vi "Periodic Tasks.vi"(8 "error in":errorcluster) -> ()   [LabVIEW 2019]
doc: "This VI runs in parallel to other tasks. It can contain as many user-defined periodic loops as you need. These can carry out PID or other sorts of timed response."
uses:
  <vilib>/Rock Robotics/WPI/ThirdParty/Sensors/navX/_TypeDefs/FRIC_navX_DeviceNumbersTypeDef.ctl
  <vilib>/Rock Robotics/WPI/DriverStation/WPI_DriverStationRobotMode2.ctl
  <vilib>/Rock Robotics/WPI/Solenoid/WPI_SolenoidValue.ctl
  <vilib>/Rock Robotics/WPI/Relay/WPI_RelayValue.ctl
  <vilib>/Rock Robotics/WPI/ThirdParty/Phoenix-LabVIEW/Motor Controller/Controls/CTRE_Phoenix_MotorControl_ControlMode.ctl
  LabVIEW_is_Under_Control.lib/Util/Toggle/Change Detect.vi
  LabVIEW_is_Under_Control.lib/Util/Toggle/Change Detect Boolean.vi
  MotorsGlobal.vi
  <vilib>/Rock Robotics/Network Tables/NT Read Number.vi
  <vilib>/Rock Robotics/WPI/Utilities/WPI_GetSetVariantRefNum.vi
  Robot Global Data.vi
  JoysticksGlobal.vi
  <vilib>/Rock Robotics/Network Tables/NT Write Number.vi
  <vilib>/Rock Robotics/WPI/Solenoid/WPI_SolenoidSetEnum.vi
  Ball Routine.ctl
  TurretMode.ctl
  <vilib>/Rock Robotics/WPI/ThirdParty/Phoenix-LabVIEW/Motor Controller/Controls/CTRE_Phoenix_MotorControl_FeedbackDevice.ctl
  Climber Routine.ctl
  <vilib>/Rock Robotics/WPI/ThirdParty/Phoenix-LabVIEW/Motor Controller/Get/CTRE_Phoenix_MotorController_GetVoltage.vi
  <vilib>/Rock Robotics/WPI/ThirdParty/Phoenix-LabVIEW/Motor Controller/Get/CTRE_Phoenix_MotorController_GetSelectedSensorData.vi
panel:
  in  "OutRoller":dbl=-0.8
  in  "OutShooter":dbl=0.6
  in  "OutConveyorRight":dbl=-0.1
  in  "OutConveyorMid":dbl=0.5
  in  "Setpoint Climber":dbl
  in  "OutIntake":dbl=0.6
  in  "OutConveyorLeft":dbl=-1.0
  out "Encoder Out":dbl
  in  "PIDs Tab":T1(tab)
  out "Current Intake":dbl
  in  "Reset Encoders":bool
  out "Current":dbl
  out "Motor Temperature":u8
  out "Current 2":dbl
  out "Motor Temperature 2":u8
  out "Current 3":dbl
  out "Motor Temperature 3":u8
  out "Current 4":dbl
  out "Motor Temperature 4":u8
  out "Current Intake 2":dbl
  out "Current Intake 3":dbl
  in  "MaxAngle":dbl
  out "LimelightX":dbl
  out "Turret PID":cluster{"Setpoint":dbl, "Process variable":dbl}(graph)
  in  "Camera Angle":dbl=7.0
  out "Distancia do Goal":dbl
  in  "Inner Goal Height":dbl=2.49
  in  "Camera Height":dbl=0.185
  in  "Minimum command":dbl=0.031
  out "Turret Out":dbl
  in  "TAGains":T2={"proportional gain (Kc)"=1.0, "integral time (Ti, min)"=0.01, "derivative time (Td, min)"=0.0} {"derivative time (Td, min)" format="%.3f"; "integral time (Ti, min)" format="%.3f"; "proportional gain (Kc)" format="%.3f"}
  in  "TADisable Range":dbl
  in  "TAIntegral Range":dbl=10000.0
  in  "TASetpoint":dbl
  in  "TARange":cluster{"output high":dbl, "output low":dbl}={"output high"=0.6, "output low"=-0.6} {"output low" format="%.2f"; "output high" format="%.2f"}
  out "Voltage":dbl
  out "Voltage Output":cluster{"Percent Output":dbl}(graph)
  out "Velocity PIDF":T3(graph)
  in  "kF":dbl=0.031
  in  "EnableFWPID":bool
  in  "FWSetpoint":dbl
  in  "P":dbl
  in  "I":dbl
  in  "D":dbl
  in  "I Zone":dbl
  # "System Tester"
  # "Sparks Max"
  # "ID-1"
  # "ID-2"
  # "ID-3"
  # "ID-4"
  # "Distance Meter"
  # "All in cm"
  # "Turret Angle PID"
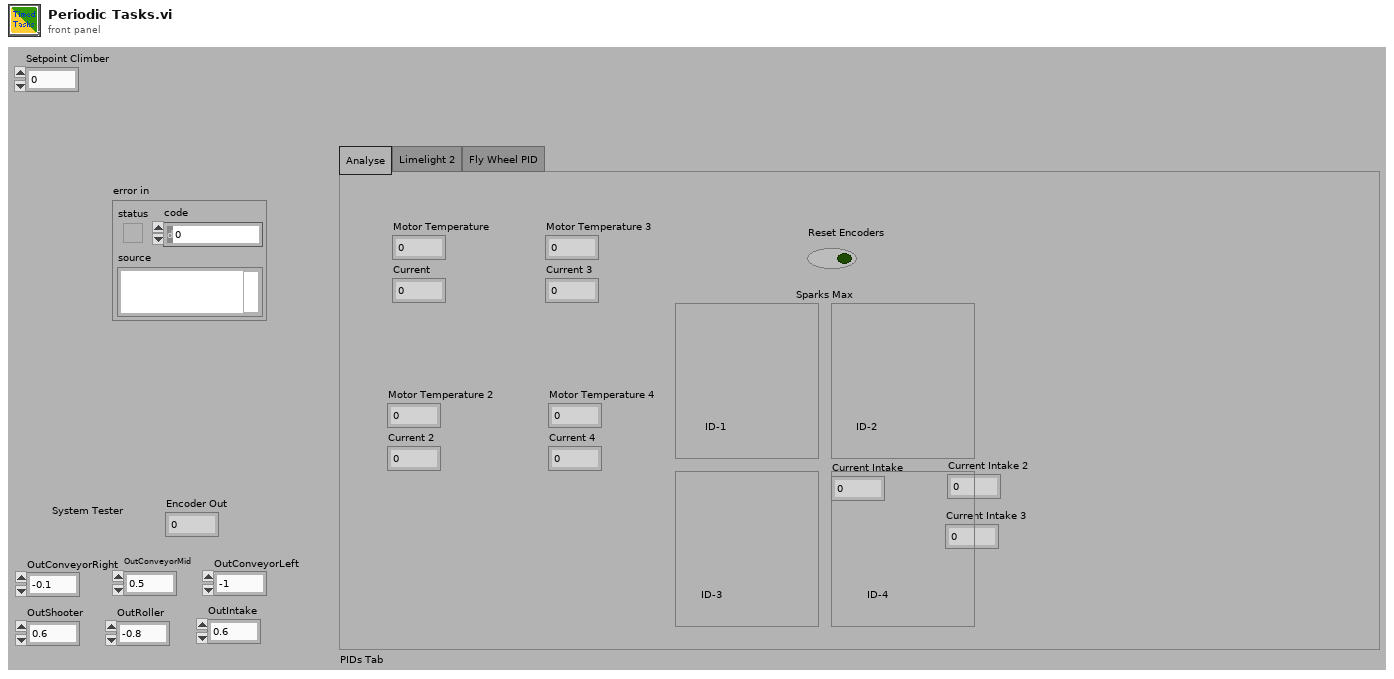
[diagram p1: front panel]
types:
  T1 = enum32{"Analyse", "Limelight 2", "Fly Wheel PID"}
  T2 = cluster{"proportional gain (Kc)":dbl, "integral time (Ti, min)":dbl, "derivative time (Td, min)":dbl}
  T3 = cluster{"FWSetpoint":dbl, "Velocity (Raw Sensor Units per 100 ms)":i32}
  T4 = typedef "WPI_EncoderDevRef.ctl" = cluster{"DevStatus":errorcluster, "EncoderIndex":T5, "CounterIndex":T6, "DistancePerCount":dbl, "Decoding Type":T7}
  T5 = typedef "FPGA_EncoderIdx.ctl" = enum8{"Enc 0", "Enc 1", "Enc 2", "Enc 3", "Enc 4", "Enc 5", "Enc 6", "Enc 7", "Invalid"}
  T6 = typedef "FPGA_CounterCtrSystemIndex.ctl" = enum8{"Ctr 0", "Ctr 1", "Ctr 2", "Ctr 3", "Ctr 4", "Ctr 5", "Ctr 6", "Ctr 7", "Invalid"}
  T7 = typedef "WPI_EncoderType.ctl" = enum16{"1x", "2x", "4x"}
  T8 = typedef "WPI_SwitchDevRef.ctl" = cluster{"DevStatus":errorcluster, "DIO Channel":T9, "CntIndex":T6, "Normally Closed":bool}
  T9 = typedef "FPGA_DIOChannel.ctl" = enum8{"DIO 0", "DIO 1", "DIO 2", "DIO 3", "DIO 4", "DIO 5", "DIO 6", "DIO 7", "DIO 8", "DIO 9", "DIO MXP 0", "DIO MXP 1", "DIO MXP 2", "DIO MXP 3", "DIO MXP 4", "DIO MXP 5", "DIO MXP 6", "DIO MXP 7", "DIO MXP 8", "DIO MXP 9", "DIO MXP 10", "DIO MXP 11", "DIO MXP 12", "DIO MXP 13", "DIO MXP 14", "DIO MXP 15", "SPI Port CS1", "SPI Port CS2", "SPI Port CS3", "SPI Port MISO", "SPI Port MOSI", "Invalid"}
  T10 = typedef "FRIC_navX_DeviceNumbersTypeDef.ctl" = enum16{"Dev0", "Dev1", "Dev2", "Dev3"}
  T11 = cluster{"Rollover":dbl, "Yaw":dbl, "Cont Yaw":dbl}
  T12 = typedef "WPI_MotorControlDeviceRef.ctl" = cluster{"DeviceStatus":errorcluster, "Type":T13, "PWM":cluster{"PWM Channel":T14, "DeadBand":T15}, "CAN":cluster{"Device Number":u8, "SetOutput VI Ref":variant, "GetOutput VI Ref":variant, "Enable VI Ref":variant, "Disable VI Ref":variant, "Data":variant}, "Invert":bool, "DIO PWM":cluster{"PWM \"Enable\" Channel":T14, "DIOChannel":T9, "PWM Rate":dbl}}
  T13 = typedef "WPI_MotorControlType.ctl" = enum16{"PWM", "CAN", "DIO PWM"}
  T14 = typedef "FPGA_DIOPWMChannel.ctl" = enum8{"PWM 0", "PWM 1", "PWM 2", "PWM 3", "PWM 4", "PWM 5", "PWM 6", "PWM 7", "PWM 8", "PWM 9", "PWM MXP 0", "PWM MXP 1", "PWM MXP 2", "PWM MXP 3", "PWM MXP 4", "PWM MXP 5", "PWM MXP 6", "PWM MXP 7", "PWM MXP 8", "PWM MXP 9", "Invalid"}
  T15 = typedef "WPI_PWMDeadband.ctl" = cluster{"Name":string, "maxPositivePwm":i32, "minPositivePwm":i32, "centerPwm":i32, "maxNegativePwm":i32, "minNegativePwm":i32, "angularRange":u16}
  T16 = typedef "WPI_JoystickDevRef.ctl" = cluster{"Device":T17}
  T17 = typedef "WPI_JoystickDeviceEnum.ctl" = enum16{"USB 0", "USB 1", "USB 2", "USB 3", "USB 4", "USB 5"}
  T18 = typedef "WPI_SolenoidDevRef.ctl" = cluster{"DevStatus":errorcluster, "Pneumatics Control Module":u8, "Forward Solenoid Channel":T19, "Reverse Solenoid Channel":T19}
  T19 = typedef "WPI_SolenoidChannel.ctl" = enum8{"Solenoid 0", "Solenoid 1", "Solenoid 2", "Solenoid 3", "Solenoid 4", "Solenoid 5", "Solenoid 6", "Solenoid 7", "Invalid"}
  T20 = typedef "WPI_RelayDevRef.ctl" = cluster{"DevStatus":errorcluster, "Relay Channel":T21, "Relay Direction":T22}
  T21 = typedef "FPGA_DIORelayChannel.ctl" = enum8{"Relay 0", "Relay 1", "Relay 2", "Relay 3", "Invalid"}
  T22 = typedef "WPI_RelayDirection.ctl" = enum16{"Both directions", "Forward only", "Reverse only"}
  T23 = typedef "WPI_RelayValue.ctl" = enum16{"Off", "On", "Forward", "Reverse"}
  T24 = typedef "WPI_SolenoidValue.ctl" = enum16{"Off", "On", "Forward", "Reverse"}
  T25 = typedef "CTRE_Phoenix_MotorControl_ControlMode.ctl" = u16
  T26 = typedef "WPI_DriverStationRobotMode2.ctl" = enum16{"Autonomous Disabled", "Autonomous Enabled", "Teleop Disabled", "Teleop Enabled", "Disconnected", "Finish", "Test Disabled", "Test Enabled", "Emergency Stopped"}
  T27 = typedef "WPI_RobotDriveDevRef.ctl" = cluster{"DevStatus":errorcluster, "Motors[]":T12[], "Square Inputs":bool, "Max Output":dbl}
  T28 = cluster{"Motors[][0]":T12, "Motors[][1]":T12, "Motors[][2]":T12, "Motors[][3]":T12, "Motors[][4]":T12, "Motors[][5]":T12, "Motors[][6]":T12, "Motors[][7]":T12, "Motors[][8]":T12}
  T29 = typedef "Climber Routine.ctl" = enum16{"Standart", "Vibrate *Lenny Face*", "Open da Boi", "Engage on the Bar!", "Pull Our Hope", "Deu por Hoje"}
  T30 = typedef "TurretMode.ctl" = enum16{"Static", "Manual", "Automatic"}
  T31 = typedef "Ball Routine.ctl" = enum16{"Standart", "Get Power Cells", "Prepare Shooter", "Shoot!"}
  T32 = typedef "CTRE_Phoenix_MotorControl_FeedbackDevice.ctl" = i8
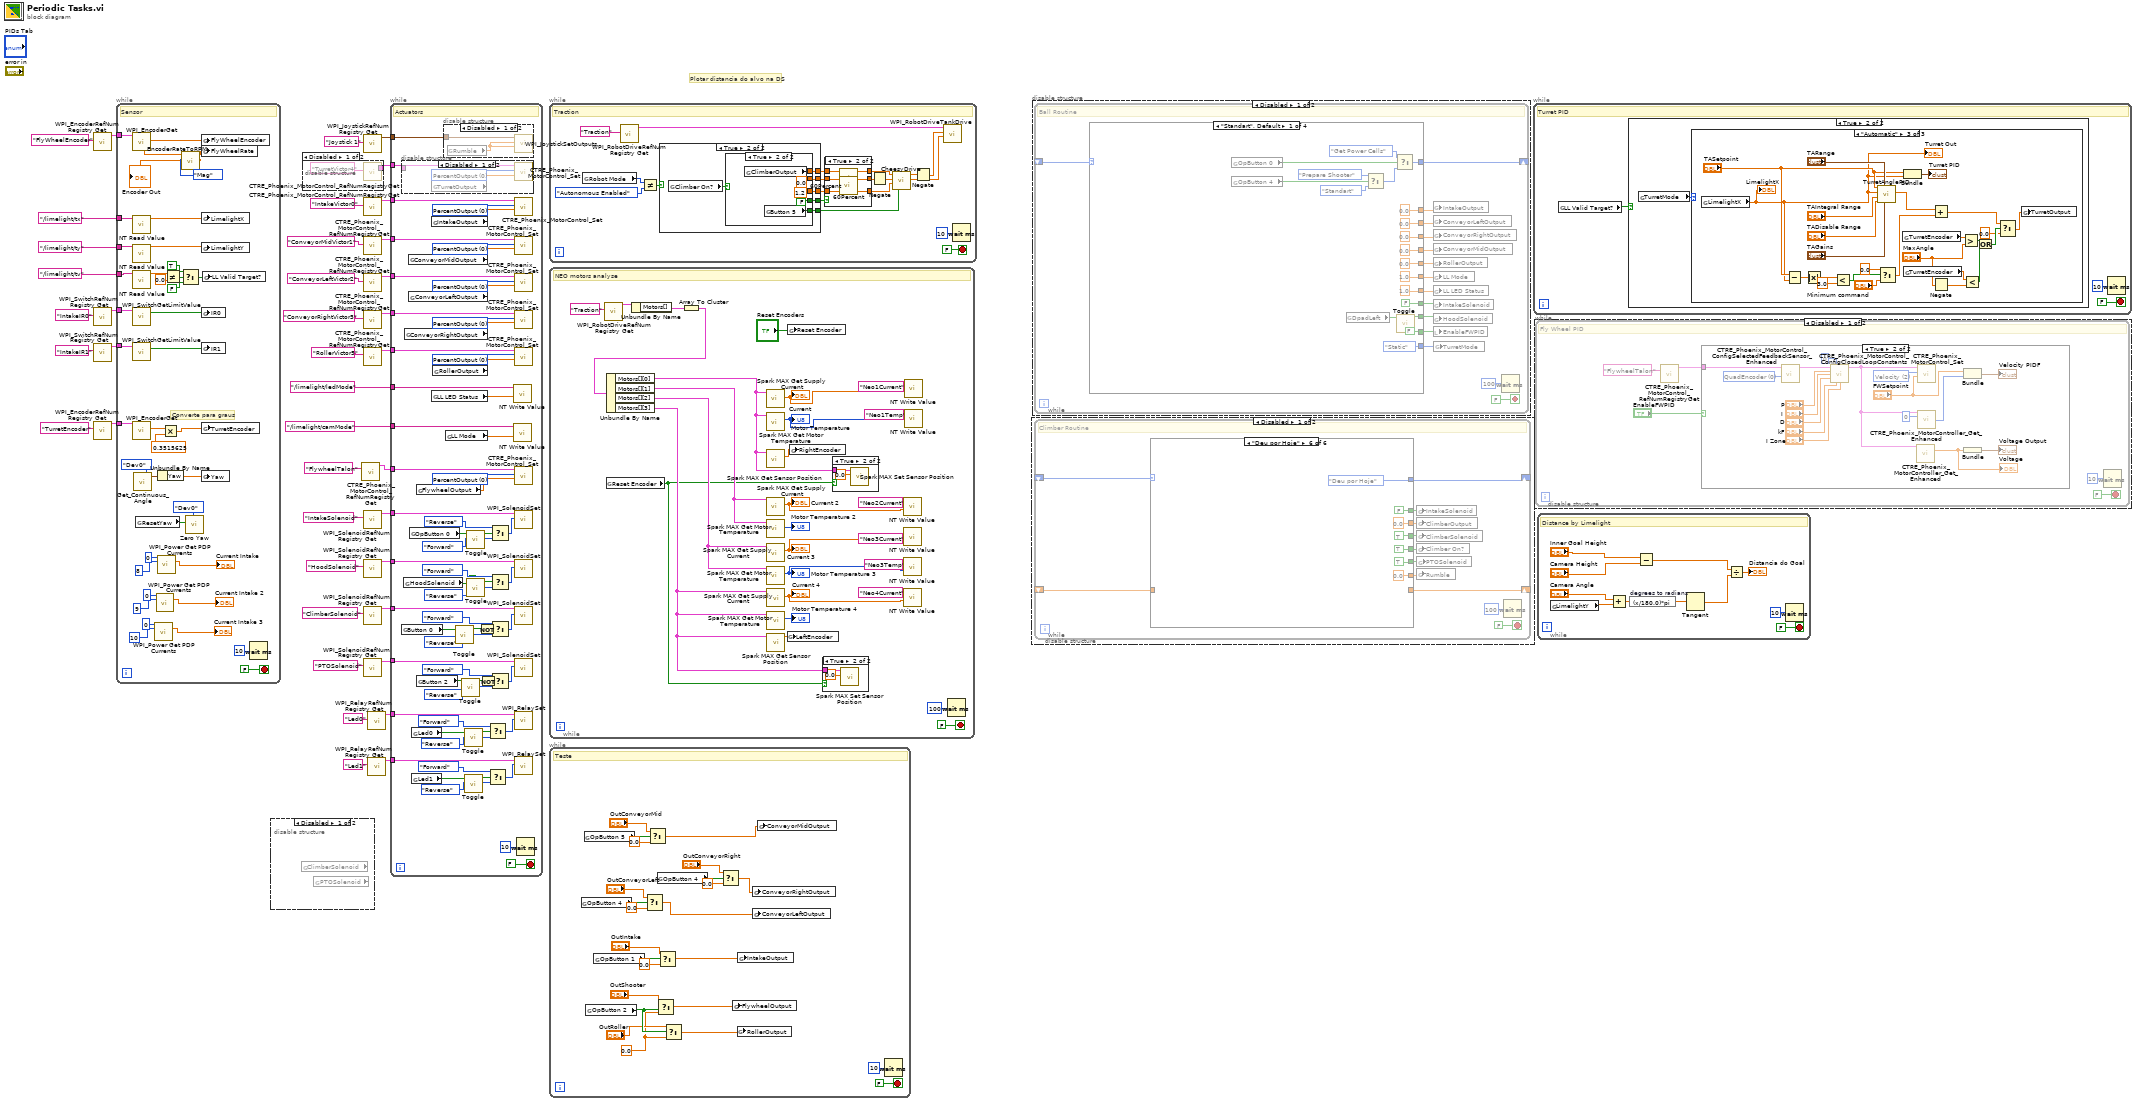
[diagram p0: block diagram]
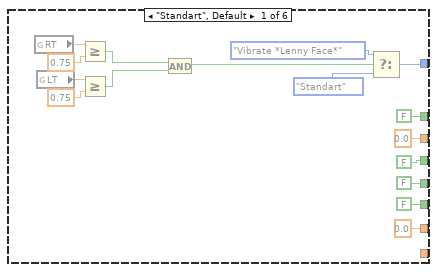
[diagram p2: hidden frame]
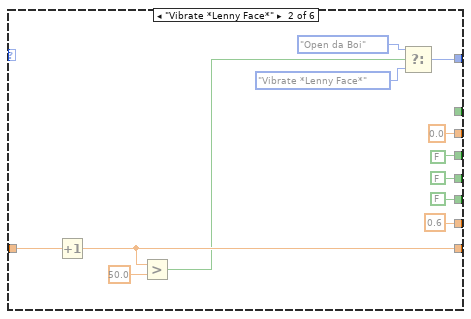
[diagram p3: hidden frame]
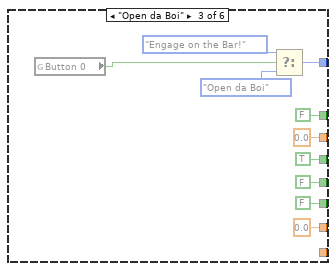
[diagram p4: hidden frame]
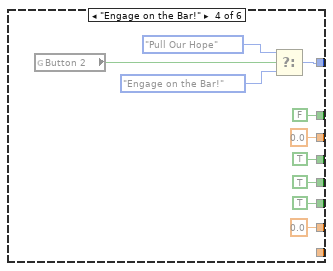
[diagram p5: hidden frame]
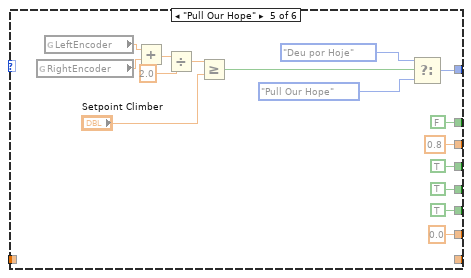
[diagram p6: hidden frame]
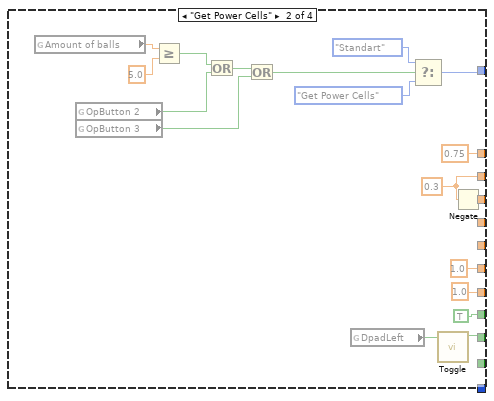
[diagram p10: hidden frame]
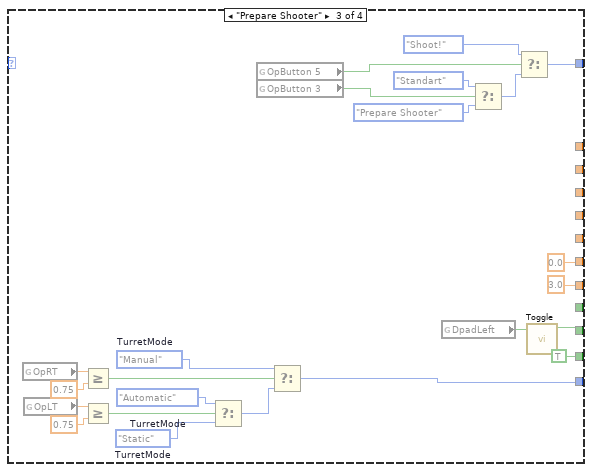
[diagram p11: hidden frame]
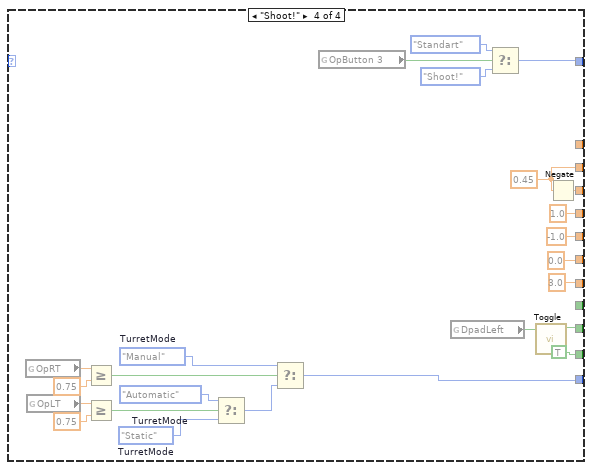
[diagram p12: hidden frame]
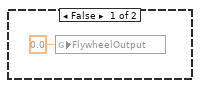
[diagram p14: hidden frame]
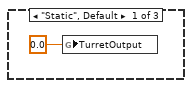
[diagram p19: hidden frame]
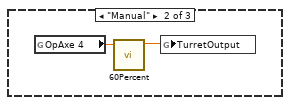
[diagram p20: hidden frame]
diagram:
  # "Plotar distancia do alvo na DS"
  n1 = call <vilib>:"WPI_EncoderRefNum Registry Get.vi"("refnum name"="FlyWheelEncoder") -> ("EncoderDevRef"=w40:T4)  [unwired: 9 in, 1 out]
  n2 = call <vilib>:"WPI_SwitchRefNum Registry Get.vi"("refnum name"="IntakeIR0") -> ("SwitchDevRef"=w23:T8)  [unwired: 9 in, 1 out]
  n3 = call <vilib>:"WPI_SwitchRefNum Registry Get.vi"("refnum name"="IntakeIR1") -> ("SwitchDevRef"=w20:T8)  [unwired: 9 in, 1 out]
  n4 = call <vilib>:"WPI_EncoderRefNum Registry Get.vi"("refnum name"="TurretEncoder") -> ("EncoderDevRef"=w15:T4)  [unwired: 9 in, 1 out]
  n5 = while {
    tunnel: w40 -> [w79]
    tunnel: "/limelight/tx" ("Name") -> [w73]
    tunnel: "/limelight/ty" ("Name") -> [w70]
    tunnel: w23 -> [w69]
    tunnel: w20 -> [w66]
    tunnel: "/limelight/tv" ("Name") -> [w65]
    tunnel: w15 -> [w58]
    stop <- FALSE stop-if-true
    # "Converte para graus"
    # "Sensor"
    n6 = call <vilib>:"WPI_EncoderGet.vi"("EncoderDevRef"=w79) -> ("Distance"=w77:dbl, "Rate"=w76:dbl)  [unwired: 5 in, 4 out]
    n7 = call-poly <vilib>:"NT Read Value.vi"("Name"=w73) -> ("Numeric"=w72:dbl)  [unwired: 9 in, 1 out]
    n8 = call-poly <vilib>:"NT Read Value.vi"("Name"=w70) -> ("Numeric"=w71:dbl)  [unwired: 9 in, 1 out]
    n9 = call-poly <vilib>:"NT Read Value.vi"("Name"=w65) -> ("Numeric"=w64:dbl)  [unwired: 9 in, 1 out]
    n10 = call <vilib>:"WPI_SwitchGetLimitValue.vi"("SwitchDevRef"=w69) -> ("Switch Pressed"=w68:bool)  [unwired: 8 in, 2 out]
    n11 = call <vilib>:"WPI_SwitchGetLimitValue.vi"("SwitchDevRef"=w66) -> ("Switch Pressed"=w67:bool)  [unwired: 8 in, 2 out]
    n12 = call <vilib>:"WPI_EncoderGet.vi"("EncoderDevRef"=w58) -> ("Distance"=w57:dbl)  [unwired: 5 in, 5 out]
    n13 = call <vilib>:"Get_Continuous_Angle.vi"("Device Number"=FRIC_navX_DeviceNumbersTypeDef."Dev0") -> ("Continuous Angle"=w53:T11)  [unwired: 10 in]
    n14 = global read "MotorsGlobal.vi" "ResetYaw"() -> (w50:bool)
    n15 = call <vilib>:"WPI_Power Get PDP Currents.vi"("Power Distribution Panel (0)"=u8 0, "PDP Channel"=10) -> ("current (A)"=→"Current Intake 3":dbl)  [unwired: 11 in, 2 out]
    n16 = call <vilib>:"WPI_Power Get PDP Currents.vi"("Power Distribution Panel (0)"=u8 0, "PDP Channel"=9) -> ("current (A)"=→"Current Intake 2":dbl)  [unwired: 11 in, 2 out]
    n17 = call <vilib>:"WPI_Power Get PDP Currents.vi"("Power Distribution Panel (0)"=u8 0, "PDP Channel"=8) -> ("current (A)"=→"Current Intake":dbl)  [unwired: 11 in, 2 out]
    n18 = Unbundle By Name(w53) -> ("Yaw"=w52:dbl)
    n19 = Multiply(x=w57, y=0.3515625) -> (x*y=w55:dbl)
    n20 = Not Equal?(x=w64, y=0.0) -> (x != y?=w62:bool)
    n21 = call "EncoderRateToRPM.vi"("Enum"=enum16{"Through Bore", "Mag"}."Mag", "EncoderRate"=w76) -> ("RPM"=→"Encoder Out":dbl, "RPS"=w75:dbl)  [unwired: 8 in]
    n22 = Select(t=TRUE, s=w62, f=FALSE) -> (s? t:f=w61:bool)
    n23 = call <vilib>:"Zero Yaw.vi"("Device Number"=FRIC_navX_DeviceNumbersTypeDef."Dev0", "Zero"=w50) -> ()  [unwired: 10 in]
    n24 = global write "MotorsGlobal.vi" "FlyWheelEncoder"(w77) -> ()
    n25 = global write "MotorsGlobal.vi" "FlyWheelRate"(w75) -> ()
    n26 = global write "MotorsGlobal.vi" "LimelightX"(w72) -> ()
    n27 = global write "MotorsGlobal.vi" "LimelightY"(w71) -> ()
    n28 = global write "MotorsGlobal.vi" "IR0"(w68) -> ()
    n29 = global write "MotorsGlobal.vi" "IR1"(w67) -> ()
    n30 = global write "MotorsGlobal.vi" "Yaw"(w52) -> ()
    n31 = global write "MotorsGlobal.vi" "TurretEncoder"(w55) -> ()
    n32 = global write "MotorsGlobal.vi" "LL Valid Target?"(w61) -> ()
    n33 = Wait (ms)(milliseconds to wait=u32 10) -> ()  [unwired: 1 out]
  }
  n34 = disable-structure shown="Disabled" {
    frame Disabled {
      n35 = global read "MotorsGlobal.vi" "ClimberSolenoid"() -> ()  [unwired: 1 out]
      n36 = global read "MotorsGlobal.vi" "PTOSolenoid"() -> ()  [unwired: 1 out]
    }
    frame Enabled {
    }
  }
  n37 = disable-structure shown="Disabled" {
    disable-tunnel: [w83 _] -> w36
    frame Disabled {
      n38 = call <vilib>:"CTRE_Phoenix_MotorControl_RefNumRegistryGet.vi"("refnum name"="TurretVictor4") -> ("PhoenixMotorControlDevRef"=w83:T12)  [unwired: 9 in, 1 out]
    }
    frame Enabled {
    }
  }
  n39 = call <vilib>:"CTRE_Phoenix_MotorControl_RefNumRegistryGet.vi"("refnum name"="FlywheelTalon") -> ("PhoenixMotorControlDevRef"=w1:T12)  [unwired: 9 in, 1 out]
  n40 = call <vilib>:"WPI_JoystickRefNum Registry Get.vi"("refnum name"="Joystick 1") -> ("JoystickDevRef"=w13:T16)  [unwired: 9 in, 1 out]
  n41 = call <vilib>:"CTRE_Phoenix_MotorControl_RefNumRegistryGet.vi"("refnum name"="IntakeVictor0") -> ("PhoenixMotorControlDevRef"=w35:T12)  [unwired: 9 in, 1 out]
  n42 = call <vilib>:"CTRE_Phoenix_MotorControl_RefNumRegistryGet.vi"("refnum name"="ConveyorMidVictor1") -> ("PhoenixMotorControlDevRef"=w34:T12)  [unwired: 9 in, 1 out]
  n43 = call <vilib>:"CTRE_Phoenix_MotorControl_RefNumRegistryGet.vi"("refnum name"="ConveyorLeftVictor2") -> ("PhoenixMotorControlDevRef"=w33:T12)  [unwired: 9 in, 1 out]
  n44 = call <vilib>:"CTRE_Phoenix_MotorControl_RefNumRegistryGet.vi"("refnum name"="ConveyorRightVictor3") -> ("PhoenixMotorControlDevRef"=w32:T12)  [unwired: 9 in, 1 out]
  n45 = call <vilib>:"CTRE_Phoenix_MotorControl_RefNumRegistryGet.vi"("refnum name"="RollerVictor5") -> ("PhoenixMotorControlDevRef"=w24:T12)  [unwired: 9 in, 1 out]
  n46 = call <vilib>:"WPI_SolenoidRefNum Registry Get.vi"("refnum name"="IntakeSolenoid") -> ("SolenoidDevRef"=w30:T18)  [unwired: 9 in, 1 out]
  n47 = call <vilib>:"WPI_SolenoidRefNum Registry Get.vi"("refnum name"="HoodSolenoid") -> ("SolenoidDevRef"=w27:T18)  [unwired: 9 in, 1 out]
  n48 = call <vilib>:"WPI_SolenoidRefNum Registry Get.vi"("refnum name"="ClimberSolenoid") -> ("SolenoidDevRef"=w26:T18)  [unwired: 9 in, 1 out]
  n49 = call <vilib>:"WPI_SolenoidRefNum Registry Get.vi"("refnum name"="PTOSolenoid") -> ("SolenoidDevRef"=w11:T18)  [unwired: 9 in, 1 out]
  n50 = call <vilib>:"WPI_RelayRefNum Registry Get.vi"("refnum name"="Led0") -> ("RelayDevRef"=w9:T20)  [unwired: 9 in, 1 out]
  n51 = call <vilib>:"WPI_RelayRefNum Registry Get.vi"("refnum name"="Led1") -> ("RelayDevRef"=w8:T20)  [unwired: 9 in, 1 out]
  n52 = while {
    tunnel: w36 -> [w145]
    tunnel: w35 -> [w144]
    tunnel: w34 -> [w143]
    tunnel: w33 -> [w142]
    tunnel: w32 -> [w141]
    tunnel: w30 -> [w140]
    tunnel: w27 -> [w131]
    tunnel: w26 -> [w130]
    tunnel: w24 -> [w125]
    tunnel: "/limelight/ledMode" ("Name") -> [w124]
    tunnel: "/limelight/camMode" ("Name") -> [w121]
    tunnel: w13 -> [w120]
    tunnel: w11 -> [w115]
    tunnel: w9 -> [w114]
    tunnel: w8 -> [w103]
    tunnel: w1 -> [w86]
    stop <- FALSE stop-if-true
    w87 = T25 0 items=["PercentOutput"=0, "Position"=1, "Velocity"=2, "Current"=3, "Follower"=5, "MotionProfile"=6, "MotionMagic"=7, "MotionProfileArc"=10, "Disabled"=15] ("Control Mode")
    w89 = T25 0 items=["PercentOutput"=0, "Position"=1, "Velocity"=2, "Current"=3, "Follower"=5, "MotionProfile"=6, "MotionMagic"=7, "MotionProfileArc"=10, "Disabled"=15] ("Control Mode")
    w95 = T25 0 items=["PercentOutput"=0, "Position"=1, "Velocity"=2, "Current"=3, "Follower"=5, "MotionProfile"=6, "MotionMagic"=7, "MotionProfileArc"=10, "Disabled"=15] ("Control Mode")
    w97 = T25 0 items=["PercentOutput"=0, "Position"=1, "Velocity"=2, "Current"=3, "Follower"=5, "MotionProfile"=6, "MotionMagic"=7, "MotionProfileArc"=10, "Disabled"=15] ("Control Mode")
    w99 = T25 0 items=["PercentOutput"=0, "Position"=1, "Velocity"=2, "Current"=3, "Follower"=5, "MotionProfile"=6, "MotionMagic"=7, "MotionProfileArc"=10, "Disabled"=15] ("Control Mode")
    w102 = T25 0 items=["PercentOutput"=0, "Position"=1, "Velocity"=2, "Current"=3, "Follower"=5, "MotionProfile"=6, "MotionMagic"=7, "MotionProfileArc"=10, "Disabled"=15] ("Control Mode")
    # "Actuators"
    n53 = disable-structure shown="Disabled" {
      disable-tunnel: w145 -> [w152 _]
      frame Disabled {
        w151 = T25 0 items=["PercentOutput"=0, "Position"=1, "Velocity"=2, "Current"=3, "Follower"=5, "MotionProfile"=6, "MotionMagic"=7, "MotionProfileArc"=10, "Disabled"=15] ("Control Mode")
        n54 = global read "MotorsGlobal.vi" "TurretOutput"() -> (w150:dbl)
        n55 = call <vilib>:"CTRE_Phoenix_MotorControl_Set.vi"("Output"=w150, "Control Mode"=w151, "PhoenixMotorControlDevRef"=w152) -> ()  [unwired: 7 in, 2 out]
      }
      frame Enabled {
      }
    }
    n56 = global read "JoysticksGlobal.vi" "Button 0"() -> (w92:bool)
    n57 = global read "MotorsGlobal.vi" "HoodSolenoid"() -> (w93:bool)
    n58 = global read "MotorsGlobal.vi" "ConveyorRightOutput"() -> (w94:dbl)
    n59 = global read "MotorsGlobal.vi" "ConveyorMidOutput"() -> (w98:dbl)
    n60 = global read "MotorsGlobal.vi" "ConveyorLeftOutput"() -> (w96:dbl)
    n61 = global read "JoysticksGlobal.vi" "OpButton 0"() -> (w100:bool)
    n62 = global read "MotorsGlobal.vi" "Led0"() -> (w109:bool)
    n63 = global read "MotorsGlobal.vi" "Led1"() -> (w108:bool)
    n64 = global read "MotorsGlobal.vi" "FlywheelOutput"() -> (w88:dbl)
    n65 = global read "JoysticksGlobal.vi" "Button 2"() -> (w91:bool)
    n66 = global read "MotorsGlobal.vi" "IntakeOutput"() -> (w101:dbl)
    n67 = global read "MotorsGlobal.vi" "LL LED Status"() -> (w123:dbl)
    n68 = global read "MotorsGlobal.vi" "RollerOutput"() -> (w90:dbl)
    n69 = disable-structure shown="Disabled" {
      disable-tunnel: w120 -> [w149 _]
      frame Disabled {
        n70 = global read "JoysticksGlobal.vi" "Rumble"() -> (w148:dbl)
        n71 = call <vilib>:"WPI_JoystickSetOutputs.vi"("Right Rumble"=w148, "Left Rumble"=w148, "JoystickDevRef"=w149) -> ()  [unwired: 7 in, 2 out]
      }
      frame Enabled {
      }
    }
    n72 = global read "MotorsGlobal.vi" "LL Mode"() -> (w122:dbl)
    n73 = call "Toggle.vi"("In"=w92) -> ("Toggled"=w126:bool)  [unwired: 10 in]
    n74 = call "Toggle.vi"("In"=w91) -> ("Toggled"=w119:bool)  [unwired: 10 in]
    n75 = call "Toggle.vi"("In"=w109) -> ("Toggled"=w113:bool)  [unwired: 10 in]
    n76 = call "Toggle.vi"("In"=w108) -> ("Toggled"=w104:bool)  [unwired: 10 in]
    n77 = call "Toggle.vi"("In"=w100) -> ("Toggled"=w136:bool)  [unwired: 10 in]
    n78 = call "Toggle.vi"("In"=w93) -> ("Toggled"=w135:bool)  [unwired: 10 in]
    n79 = Not(x=w126) -> (.not. x?=w85:bool)
    n80 = Not(x=w119) -> (.not. x?=w84:bool)
    n81 = Select(t=WPI_RelayValue."Forward" ("RelayValue"), s=w113, f=WPI_RelayValue."Reverse" ("RelayValue")) -> (s? t:f=w112:T23)
    n82 = Select(t=WPI_RelayValue."Forward" ("RelayValue"), s=w104, f=WPI_RelayValue."Reverse" ("RelayValue")) -> (s? t:f=w105:T23)
    n83 = Select(t=WPI_SolenoidValue."Reverse" ("Value"), s=w136, f=WPI_SolenoidValue."Forward" ("Value")) -> (s? t:f=w138:T24)
    n84 = Select(t=WPI_SolenoidValue."Forward" ("Value"), s=w135, f=WPI_SolenoidValue."Reverse" ("Value")) -> (s? t:f=w133:T24)
    n85 = Select(t=WPI_SolenoidValue."Forward" ("Value"), s=w85, f=WPI_SolenoidValue."Reverse" ("Value")) -> (s? t:f=w128:T24)
    n86 = Select(t=WPI_SolenoidValue."Forward" ("Value"), s=w84, f=WPI_SolenoidValue."Reverse" ("Value")) -> (s? t:f=w117:T24)
    n87 = call-poly <vilib>:"NT Write Value.vi"("Numeric"=w123, "Name"=w124) -> ()  [unwired: 9 in, 1 out]
    n88 = call-poly <vilib>:"NT Write Value.vi"("Numeric"=w122, "Name"=w121) -> ()  [unwired: 9 in, 1 out]
    n89 = call <vilib>:"CTRE_Phoenix_MotorControl_Set.vi"("Output"=w101, "Control Mode"=w102, "PhoenixMotorControlDevRef"=w144) -> ()  [unwired: 7 in, 2 out]
    n90 = call <vilib>:"CTRE_Phoenix_MotorControl_Set.vi"("Output"=w98, "Control Mode"=w99, "PhoenixMotorControlDevRef"=w143) -> ()  [unwired: 7 in, 2 out]
    n91 = call <vilib>:"CTRE_Phoenix_MotorControl_Set.vi"("Output"=w96, "Control Mode"=w97, "PhoenixMotorControlDevRef"=w142) -> ()  [unwired: 7 in, 2 out]
    n92 = call <vilib>:"CTRE_Phoenix_MotorControl_Set.vi"("Output"=w94, "Control Mode"=w95, "PhoenixMotorControlDevRef"=w141) -> ()  [unwired: 7 in, 2 out]
    n93 = call <vilib>:"CTRE_Phoenix_MotorControl_Set.vi"("Output"=w90, "Control Mode"=w89, "PhoenixMotorControlDevRef"=w125) -> ()  [unwired: 7 in, 2 out]
    n94 = call <vilib>:"CTRE_Phoenix_MotorControl_Set.vi"("Output"=w88, "Control Mode"=w87, "PhoenixMotorControlDevRef"=w86) -> ()  [unwired: 7 in, 2 out]
    n95 = call-poly <vilib>:"WPI_SolenoidSet.vi"("Value"=w138, "SolenoidDevRef"=w140) -> ()  [unwired: 8 in, 2 out]
    n96 = call-poly <vilib>:"WPI_SolenoidSet.vi"("Value"=w133, "SolenoidDevRef"=w131) -> ()  [unwired: 8 in, 2 out]
    n97 = call-poly <vilib>:"WPI_SolenoidSet.vi"("Value"=w128, "SolenoidDevRef"=w130) -> ()  [unwired: 8 in, 2 out]
    n98 = call-poly <vilib>:"WPI_SolenoidSet.vi"("Value"=w117, "SolenoidDevRef"=w115) -> ()  [unwired: 8 in, 2 out]
    n99 = call <vilib>:"WPI_RelaySet.vi"("RelayValue"=w112, "RelayDevRef"=w114) -> ()  [unwired: 8 in, 2 out]
    n100 = call <vilib>:"WPI_RelaySet.vi"("RelayValue"=w105, "RelayDevRef"=w103) -> ()  [unwired: 8 in, 2 out]
    n101 = Wait (ms)(milliseconds to wait=u32 10) -> ()  [unwired: 1 out]
  }
  n102 = while {
    stop <- FALSE stop-if-true
    # "Traction"
    n103 = global read "Robot Global Data.vi" "Robot Mode"() -> (w156:T26)
    n104 = call <vilib>:"WPI_RobotDriveRefNum Registry Get.vi"("refnum name"="Traction") -> ("RobotDriveDevRef"=w169:T27)  [unwired: 9 in, 1 out]
    n105 = Not Equal?(x=w156, y=WPI_DriverStationRobotMode2."Autonomous Enabled") -> (x != y?=w154:bool)
    n106 = case shown="True" w154 {
      tunnel: [w176 w182] -> w162
      tunnel: [w175 w181] -> w161
      tunnel: [1.0 ("Sensitivty") w180] -> w159
      tunnel: [FALSE ("Button 4") w179] -> w158
      tunnel: [TRUE ("Button 5") w178] -> w157
      frame False {
        n107 = global read "JoysticksGlobal.vi" "AutoAxe1"() -> (w176:dbl)
        n108 = global read "JoysticksGlobal.vi" "AutoAxe4"() -> (w175:dbl)
      }
      frame True {
        n109 = global read "MotorsGlobal.vi" "Climber On?"() -> (w177:bool)
        n110 = case shown="True" w177 {
          tunnel: [w187 w189] -> w182
          tunnel: [w186 0.0 ("Axe 4")] -> w181
          tunnel: [1.2 ("Sensitivty") 1.2 ("Sensitivty")] -> w180
          tunnel: [w184 FALSE ("Button 4")] -> w179
          tunnel: [w183 w191] -> w178
          frame False {
            n111 = global read "JoysticksGlobal.vi" "Button 4"() -> (w184:bool)
            n112 = global read "JoysticksGlobal.vi" "Button 5"() -> (w183:bool)
            n113 = global read "JoysticksGlobal.vi" "Axe 1"() -> (w187:dbl)
            n114 = global read "JoysticksGlobal.vi" "Axe 4"() -> (w186:dbl)
          }
          frame True {
            n115 = global read "MotorsGlobal.vi" "ClimberOutput"() -> (w189:dbl)
            n116 = global read "JoysticksGlobal.vi" "Button 5"() -> (w191:bool)
          }
        }
      }
    }
    n117 = case shown="True" w158 {
      tunnel: [w194 w200] -> w167
      tunnel: [w195 w199] -> w153
      tunnel: w162 -> [w195 w197]
      tunnel: w161 -> [w194 w198]
      tunnel: [w193 w196] -> w160
      tunnel: w159 -> [w193 w196]
      frame False {
      }
      frame True {
        n118 = call "60Percent.vi"("In"=w197) -> ("Out"=w199:dbl)  [unwired: 9 in]
        n119 = call "60Percent.vi"("In"=w198) -> ("Out"=w200:dbl)  [unwired: 9 in]
      }
    }
    n120 = Negate(x=w167) -> (-x=w163:dbl)
    n121 = call "CheesyDrive.vi"("Quickturn"=w157, "Sensitivty"=w160, "Wheel"=w163, "Throttle"=w153) -> ("Right PWM"=w164:dbl, "Left PWM"=w166:dbl)  [unwired: 6 in]
    n122 = Negate(x=w166) -> (-x=w165:dbl)
    n123 = call <vilib>:"WPI_RobotDriveTankDrive.vi"("Right axis value"=w164, "Left axis value"=w165, "RobotDriveDevRef"=w169) -> ()  [unwired: 6 in, 3 out]
    n124 = Wait (ms)(milliseconds to wait=u32 10) -> ()  [unwired: 1 out]
  }
  n125 = while {
    stop <- FALSE stop-if-true
    # "NEO motors analyse"
    n126 = call <vilib>:"WPI_RobotDriveRefNum Registry Get.vi"("refnum name"="Traction") -> ("RobotDriveDevRef"=w227:T27)  [unwired: 9 in, 1 out]
    n127 = global read "MotorsGlobal.vi" "Reset Encoder"() -> (w204:bool)
    n128 = Unbundle By Name(w227) -> ("Motors[]"=w226:T12[])
    n129 = Array To Cluster(array=w226) -> (cluster=w221:T28)
    n130 = Unbundle By Name(w221) -> ("Motors[][0]"=w206:T12, "Motors[][1]"=w220:T12, "Motors[][2]"=w219:T12, "Motors[][3]"=w205:T12)
    n131 = call <vilib>:"Spark MAX Get Supply Current.vi"("MotorControlDevRef in"=w206) -> ("Current"=w217:dbl)  [unwired: 7 in, 3 out]
    "Current" <- w217
    n132 = call <vilib>:"Spark MAX Get Motor Temperature.vi"("MotorControlDevRef in"=w206) -> ("Motor Temperature"=w215:u8)  [unwired: 7 in, 3 out]
    "Motor Temperature" <- w215
    n133 = call <vilib>:"Spark MAX Get Sensor Position.vi"("MotorControlDevRef in"=w206) -> ("Sensor Position"=w203:dbl)  [unwired: 7 in, 3 out]
    n134 = call <vilib>:"Spark MAX Get Supply Current.vi"("MotorControlDevRef in"=w220) -> ("Current"=w214:dbl)  [unwired: 7 in, 3 out]
    "Current 2" <- w214
    n135 = call <vilib>:"Spark MAX Get Motor Temperature.vi"("MotorControlDevRef in"=w220) -> ("Motor Temperature"=→"Motor Temperature 2":u8)  [unwired: 7 in, 3 out]
    n136 = call <vilib>:"Spark MAX Get Supply Current.vi"("MotorControlDevRef in"=w219) -> ("Current"=w213:dbl)  [unwired: 7 in, 3 out]
    "Current 3" <- w213
    n137 = call <vilib>:"Spark MAX Get Motor Temperature.vi"("MotorControlDevRef in"=w219) -> ("Motor Temperature"=w212:u8)  [unwired: 7 in, 3 out]
    "Motor Temperature 3" <- w212
    n138 = call <vilib>:"Spark MAX Get Supply Current.vi"("MotorControlDevRef in"=w205) -> ("Current"=w211:dbl)  [unwired: 7 in, 3 out]
    "Current 4" <- w211
    n139 = call <vilib>:"Spark MAX Get Motor Temperature.vi"("MotorControlDevRef in"=w205) -> ("Motor Temperature"=→"Motor Temperature 4":u8)  [unwired: 7 in, 3 out]
    n140 = call <vilib>:"Spark MAX Get Sensor Position.vi"("MotorControlDevRef in"=w205) -> ("Sensor Position"=w202:dbl)  [unwired: 7 in, 3 out]
    n141 = global write "MotorsGlobal.vi" "LeftEncoder"(w202) -> ()
    n142 = global write "MotorsGlobal.vi" "Reset Encoder"("Reset Encoders") -> ()
    n143 = global write "MotorsGlobal.vi" "RightEncoder"(w203) -> ()
    n144 = case shown="True" w204 {
      tunnel: w205 -> [_ w230]
      frame False {
      }
      frame True {
        n145 = call <vilib>:"Spark MAX Set Sensor Position.vi"("Position"=0.0, "MotorControlDeviceRef"=w230) -> ()  [unwired: 8 in, 2 out]
      }
    }
    n146 = case shown="True" w204 {
      tunnel: w206 -> [_ w232]
      frame False {
      }
      frame True {
        n147 = call <vilib>:"Spark MAX Set Sensor Position.vi"("Position"=0.0, "MotorControlDeviceRef"=w232) -> ()  [unwired: 8 in, 2 out]
      }
    }
    n148 = call-poly <vilib>:"NT Write Value.vi"("Numeric"=w214, "Name"="Neo2Current") -> ()  [unwired: 9 in, 1 out]
    n149 = call-poly <vilib>:"NT Write Value.vi"("Numeric"=w213, "Name"="Neo3Current") -> ()  [unwired: 9 in, 1 out]
    n150 = call-poly <vilib>:"NT Write Value.vi"("Numeric"=w212, "Name"="Neo3Temp") -> ()  [unwired: 9 in, 1 out]
    n151 = call-poly <vilib>:"NT Write Value.vi"("Numeric"=w211, "Name"="Neo4Current") -> ()  [unwired: 9 in, 1 out]
    n152 = call-poly <vilib>:"NT Write Value.vi"("Numeric"=w217, "Name"="Neo1Current") -> ()  [unwired: 9 in, 1 out]
    n153 = call-poly <vilib>:"NT Write Value.vi"("Numeric"=w215, "Name"="Neo1Temp") -> ()  [unwired: 9 in, 1 out]
    n154 = Wait (ms)(milliseconds to wait=u32 100) -> ()  [unwired: 1 out]
  }
  n155 = while {
    stop <- FALSE stop-if-true
    w233 = 0.0 ("f")
    # "Teste"
    n156 = global read "JoysticksGlobal.vi" "OpButton 4"() -> (w254:bool)
    n157 = global read "JoysticksGlobal.vi" "OpButton 5"() -> (w246:bool)
    n158 = global read "JoysticksGlobal.vi" "OpButton 2"() -> (w236:bool)
    n159 = global read "JoysticksGlobal.vi" "OpButton 1"() -> (w250:bool)
    n160 = Select(t="OutConveyorLeft", s=w254, f=0.0) -> (s? t:f=w243:dbl)
    n161 = Select(t="OutConveyorMid", s=w246, f=0.0) -> (s? t:f=w245:dbl)
    n162 = global read "JoysticksGlobal.vi" "OpButton 4"() -> (w240:bool)
    n163 = Select(t="OutShooter", s=w236, f=w233) -> (s? t:f=w238:dbl)
    n164 = Select(t="OutIntake", s=w250, f=0.0) -> (s? t:f=w248:dbl)
    n165 = Select(t="OutRoller", s=w236, f=w233) -> (s? t:f=w235:dbl)
    n166 = Select(t="OutConveyorRight", s=w240, f=0.0) -> (s? t:f=w239:dbl)
    n167 = global write "MotorsGlobal.vi" "FlywheelOutput"(w238) -> ()
    n168 = global write "MotorsGlobal.vi" "RollerOutput"(w235) -> ()
    n169 = global write "MotorsGlobal.vi" "IntakeOutput"(w248) -> ()
    n170 = global write "MotorsGlobal.vi" "ConveyorRightOutput"(w239) -> ()
    n171 = global write "MotorsGlobal.vi" "ConveyorLeftOutput"(w243) -> ()
    n172 = global write "MotorsGlobal.vi" "ConveyorMidOutput"(w245) -> ()
    n173 = Wait (ms)(milliseconds to wait=u32 10) -> ()  [unwired: 1 out]
  }
  n174 = disable-structure shown="Disabled" {
    frame Disabled {
      n175 = while {
        shift-right: [w264] -> _
        shift-left: _ -> [w263]
        shift-right: [w260] -> _
        shift-left: _ -> [w261]
        stop <- FALSE stop-if-true
        # "Climber Routine"
        n176 = case shown="\"Deu por Hoje\"" w263 {
          tunnel: [FALSE FALSE FALSE TRUE TRUE TRUE] -> w259
          tunnel: [0.0 0.0 0.0 0.0 0.8 0.0] -> w266
          tunnel: [FALSE FALSE TRUE TRUE TRUE TRUE] -> w265
          tunnel: [w281 w295 w302 w309 w322 Climber_Routine."Deu por Hoje"] -> w264
          tunnel: [0.0 0.6 0.0 0.0 0.0 0.0] -> w262
          tunnel: w261 -> [_ w294 _ _ _ _]
          tunnel: [_ w293 _ _ _ _] -> w260
          tunnel: [FALSE FALSE FALSE TRUE TRUE TRUE] -> w258
          tunnel: [FALSE _ FALSE FALSE FALSE FALSE] -> w257
          frame "Standart", Default {
            n177 = global read "JoysticksGlobal.vi" "RT"() -> (w274:dbl)
            n178 = global read "JoysticksGlobal.vi" "LT"() -> (w273:dbl)
            n179 = Greater Or Equal?(x=w274, y=0.75) -> (x >= y?=w270:bool)
            n180 = Greater Or Equal?(x=w273, y=0.75) -> (x >= y?=w269:bool)
            n181 = And(x=w270, y=w269) -> (x .and. y?=w283:bool)
            n182 = Select(t=Climber_Routine."Vibrate *Lenny Face*", s=w283, f=Climber_Routine."Standart") -> (s? t:f=w281:T29)
          }
          frame "Vibrate *Lenny Face*" {
            n183 = Increment(x=w294) -> (x+1=w293:dbl)
            n184 = Greater?(x=w293, y=50.0) -> (0:w291:bool)
            n185 = Select(t=Climber_Routine."Open da Boi", s=w291, f=Climber_Routine."Vibrate *Lenny Face*") -> (s? t:f=w295:T29)
          }
          frame "Open da Boi" {
            n186 = global read "JoysticksGlobal.vi" "Button 0"() -> (w299:bool)
            n187 = Select(t=Climber_Routine."Engage on the Bar!", s=w299, f=Climber_Routine."Open da Boi") -> (s? t:f=w302:T29)
          }
          frame "Engage on the Bar!" {
            n188 = global read "JoysticksGlobal.vi" "Button 2"() -> (w310:bool)
            n189 = Select(t=Climber_Routine."Pull Our Hope", s=w310, f=Climber_Routine."Engage on the Bar!") -> (s? t:f=w309:T29)
          }
          frame "Pull Our Hope" {
            n190 = global read "MotorsGlobal.vi" "RightEncoder"() -> (w319:dbl)
            n191 = global read "MotorsGlobal.vi" "LeftEncoder"() -> (w318:dbl)
            n192 = Add(x=w318, y=w319) -> (x+y=w328:dbl)
            n193 = Divide(x=w328, y=2.0) -> (x/y=w326:dbl)
            n194 = Greater Or Equal?(x=w326, y="Setpoint Climber") -> (x >= y?=w321:bool)
            n195 = Select(t=Climber_Routine."Deu por Hoje", s=w321, f=Climber_Routine."Pull Our Hope") -> (s? t:f=w322:T29)
          }
          frame "Deu por Hoje" {
          }
        }
        n196 = global write "MotorsGlobal.vi" "IntakeSolenoid"(w257) -> ()
        n197 = global write "MotorsGlobal.vi" "ClimberOutput"(w266) -> ()
        n198 = global write "MotorsGlobal.vi" "ClimberSolenoid"(w265) -> ()
        n199 = global write "MotorsGlobal.vi" "Climber On?"(w259) -> ()
        n200 = global write "JoysticksGlobal.vi" "Rumble"(w262) -> ()
        n201 = global write "MotorsGlobal.vi" "PTOSolenoid"(w258) -> ()
        n202 = Wait (ms)(milliseconds to wait=u32 100) -> ()  [unwired: 1 out]
      }
    }
    frame Enabled {
    }
  }
  n203 = disable-structure shown="Disabled" {
    frame Disabled {
      n204 = while {
        shift-right: [w351] -> _
        shift-left: _ -> [w352]
        stop <- FALSE stop-if-true
        # "Ball Routine"
        n205 = case shown="\"Standart\", Default" w352 {
          tunnel: [w373 w383 w399 w420] -> w351
          tunnel: [0.0 0.75 _ _] -> w350
          tunnel: [0.0 _ _ -1.0] -> w349
          tunnel: [0.0 w375 _ w416] -> w348
          tunnel: [0.0 w374 _ w415] -> w347
          tunnel: [0.0 _ _ 1.0] -> w346
          tunnel: [FALSE ("IntakeSolenoid") TRUE ("IntakeSolenoid") _ _] -> w345
          tunnel: [w359 w389 w402 w426] -> w344
          tunnel: [TurretMode."Static" ("TurretMode") _ w403 w428] -> w343
          tunnel: [FALSE ("IntakeSolenoid") _ TRUE ("IntakeSolenoid") TRUE ("IntakeSolenoid")] -> w342
          tunnel: [1.0 1.0 3.0 3.0] -> w341
          tunnel: [1.0 1.0 0.0 0.0] -> w340
          frame "Standart", Default {
            n206 = global read "JoysticksGlobal.vi" "OpButton 0"() -> (w361:bool)
            n207 = global read "JoysticksGlobal.vi" "OpButton 4"() -> (w362:bool)
            n208 = global read "JoysticksGlobal.vi" "DpadLeft"() -> (w360:bool)
            n209 = Select(t=Ball_Routine."Prepare Shooter", s=w362, f=Ball_Routine."Standart") -> (s? t:f=w365:T31)
            n210 = Select(t=Ball_Routine."Get Power Cells", s=w361, f=w365) -> (s? t:f=w373:T31)
            n211 = call "Toggle.vi"("In"=w360) -> ("Toggled"=w359:bool)  [unwired: 10 in]
          }
          frame "Get Power Cells" {
            w375 = 0.3
            n212 = global read "MotorsGlobal.vi" "Amount of balls"() -> (w387:dbl)
            n213 = global read "JoysticksGlobal.vi" "OpButton 2"() -> (w384:bool)
            n214 = global read "JoysticksGlobal.vi" "OpButton 3"() -> (w380:bool)
            n215 = Greater Or Equal?(x=w387, y=5.0) -> (x >= y?=w385:bool)
            n216 = Or(x=w385, y=w384) -> (x .or. y?=w379:bool)
            n217 = Or(x=w379, y=w380) -> (x .or. y?=w378:bool)
            n218 = global read "JoysticksGlobal.vi" "DpadLeft"() -> (w390:bool)
            n219 = Select(t=Ball_Routine."Standart", s=w378, f=Ball_Routine."Get Power Cells") -> (s? t:f=w383:T31)
            n220 = call "Toggle.vi"("In"=w390) -> ("Toggled"=w389:bool)  [unwired: 10 in]
            n221 = Negate(x=w375) -> (-x=w374:dbl)
          }
          frame "Prepare Shooter" {
            w408 = TurretMode."Manual"  # TurretMode
            w406 = TurretMode."Automatic"  # TurretMode
            w407 = TurretMode."Static"  # TurretMode
            n222 = global read "JoysticksGlobal.vi" "OpRT"() -> (w411:dbl)
            n223 = global read "JoysticksGlobal.vi" "OpLT"() -> (w410:dbl)
            n224 = Greater Or Equal?(x=w411, y=0.75) -> (x >= y?=w413:bool)
            n225 = Greater Or Equal?(x=w410, y=0.75) -> (x >= y?=w412:bool)
            n226 = Select(t=w406, s=w412, f=w407) -> (s? t:f=w409:T30)
            n227 = global read "JoysticksGlobal.vi" "OpButton 5"() -> (w398:bool)
            n228 = global read "JoysticksGlobal.vi" "OpButton 3"() -> (w396:bool)
            n229 = Select(t=w408, s=w413, f=w409) -> (s? t:f=w403:T30)
            n230 = global read "JoysticksGlobal.vi" "DpadLeft"() -> (w414:bool)
            n231 = Select(t=Ball_Routine."Standart", s=w396, f=Ball_Routine."Prepare Shooter") -> (s? t:f=w397:T31)
            n232 = Select(t=Ball_Routine."Shoot!", s=w398, f=w397) -> (s? t:f=w399:T31)
            n233 = call "Toggle.vi"("In"=w414) -> ("Toggled"=w402:bool)  [unwired: 10 in]
          }
          frame "Shoot!" {
            w416 = 0.45
            w433 = TurretMode."Manual"  # TurretMode
            w431 = TurretMode."Automatic"  # TurretMode
            w432 = TurretMode."Static"  # TurretMode
            n234 = global read "JoysticksGlobal.vi" "OpRT"() -> (w436:dbl)
            n235 = global read "JoysticksGlobal.vi" "OpLT"() -> (w435:dbl)
            n236 = Greater Or Equal?(x=w436, y=0.75) -> (x >= y?=w438:bool)
            n237 = Greater Or Equal?(x=w435, y=0.75) -> (x >= y?=w437:bool)
            n238 = Select(t=w431, s=w437, f=w432) -> (s? t:f=w434:T30)
            n239 = Select(t=w433, s=w438, f=w434) -> (s? t:f=w428:T30)
            n240 = global read "JoysticksGlobal.vi" "OpButton 3"() -> (w422:bool)
            n241 = global read "JoysticksGlobal.vi" "DpadLeft"() -> (w427:bool)
            n242 = Select(t=Ball_Routine."Standart", s=w422, f=Ball_Routine."Shoot!") -> (s? t:f=w420:T31)
            n243 = call "Toggle.vi"("In"=w427) -> ("Toggled"=w426:bool)  [unwired: 10 in]
            n244 = Negate(x=w416) -> (-x=w415:dbl)
          }
        }
        n245 = global write "MotorsGlobal.vi" "IntakeOutput"(w350) -> ()
        n246 = global write "MotorsGlobal.vi" "ConveyorLeftOutput"(w348) -> ()
        n247 = global write "MotorsGlobal.vi" "ConveyorRightOutput"(w347) -> ()
        n248 = global write "MotorsGlobal.vi" "ConveyorMidOutput"(w346) -> ()
        n249 = global write "MotorsGlobal.vi" "RollerOutput"(w349) -> ()
        n250 = global write "MotorsGlobal.vi" "LL Mode"(w340) -> ()
        n251 = global write "MotorsGlobal.vi" "LL LED Status"(w341) -> ()
        n252 = global write "MotorsGlobal.vi" "IntakeSolenoid"(w345) -> ()
        n253 = global write "MotorsGlobal.vi" "HoodSolenoid"(w344) -> ()
        n254 = local write "EnableFWPID"(w342) -> ()
        n255 = global write "MotorsGlobal.vi" "TurretMode"(w343) -> ()
        n256 = Wait (ms)(milliseconds to wait=u32 100) -> ()  [unwired: 1 out]
      }
    }
    frame Enabled {
    }
  }
  n257 = while {
    stop <- FALSE stop-if-true
    # "Turret PID"
    n258 = global read "MotorsGlobal.vi" "LL Valid Target?"() -> (w439:bool)
    n259 = case shown="True" w439 {
      frame False {
      }
      frame True {
        n260 = global read "MotorsGlobal.vi" "TurretMode"() -> (w442:T30)
        n261 = case shown="\"Automatic\"" w442 {
          frame "Static", Default {
            n262 = global write "MotorsGlobal.vi" "TurretOutput"(0.0 ("FlywheelOutput")) -> ()
          }
          frame "Manual" {
            n263 = global read "JoysticksGlobal.vi" "OpAxe 4"() -> (w445:dbl)
            n264 = call "60Percent.vi"("In"=w445) -> ("Out"=w444:dbl)  [unwired: 9 in]
            n265 = global write "MotorsGlobal.vi" "TurretOutput"(w444) -> ()
          }
          frame "Automatic" {
            n266 = global read "MotorsGlobal.vi" "LimelightX"() -> (w463:dbl)
            "Turret Out" <- w463
            "LimelightX" <- w463
            n267 = Subtract(x="TASetpoint", y=w463) -> (x-y=w462:dbl)
            n268 = Absolute Value(x=w462) -> (abs(x)=w461:dbl)
            n269 = Less?(x=w461, y=3.0) -> (x < y?=w459:bool)
            n270 = call "TurretAnglePID.vi"("TAGains"="TAGains", "TARange"="TARange", "TADisable Range"="TADisable Range", "TAIntegral Range"="TAIntegral Range", "TAProcess variable"=w463, "TASetpoint"="TASetpoint") -> ("TAoutput"=w465:dbl)  [unwired: 5 in]
            n271 = Select(t=0.0, s=w459, f="Minimum command") -> (s? t:f=w456:dbl)
            n272 = global read "MotorsGlobal.vi" "TurretEncoder"() -> (w455:dbl)
            n273 = Bundle("TASetpoint"="TASetpoint", "LimelightX"=w463) -> (→"Turret PID":cluster{"TASetpoint":dbl, "LimelightX":dbl})  [unwired: 1 in]
            n274 = global read "MotorsGlobal.vi" "TurretEncoder"() -> (w451:dbl)
            n275 = Add(x=w465, y=w456) -> (x+y=w448:dbl)
            n276 = Negate(x="MaxAngle") -> (-x=w450:dbl)
            n277 = Greater?(x=w455, y="MaxAngle") -> (0:w454:bool)
            n278 = Less?(x=w451, y=w450) -> (x < y?=w452:bool)
            n279 = Or(x=w454, y=w452) -> (x .or. y?=w447:bool)
            n280 = Select(t=w448, s=w447, f=0.0) -> (s? t:f=w449:dbl)
            n281 = global write "MotorsGlobal.vi" "TurretOutput"(w449) -> ()
          }
        }
      }
    }
    n282 = Wait (ms)(milliseconds to wait=u32 10) -> ()  [unwired: 1 out]
  }
  n283 = disable-structure shown="Disabled" {
    frame Disabled {
      n284 = while {
        stop <- FALSE stop-if-true
        # "Fly Wheel PID"
        n285 = call <vilib>:"CTRE_Phoenix_MotorControl_RefNumRegistryGet.vi"("refnum name"="FlywheelTalon") -> ("PhoenixMotorControlDevRef"=w471:T12)  [unwired: 9 in, 1 out]
        n286 = case shown="True" "EnableFWPID" {
          tunnel: w471 -> [_ w493]
          frame False {
            n287 = global write "MotorsGlobal.vi" "FlywheelOutput"(0.0 ("FlywheelOutput")) -> ()
          }
          frame True {
            w484 = T25 2 items=["PercentOutput"=0, "Position"=1, "Velocity"=2, "Current"=3, "Follower"=5, "MotionProfile"=6, "MotionMagic"=7, "MotionProfileArc"=10, "Disabled"=15] ("Control Mode")
            w492 = T32 0 items=["QuadEncoder"=0, "Analog"=2, "Tachometer"=4, "Pulse Width Encoded Position"=8, "Sensor Sum (S0 + S1)"=9, "Sensor Difference (D0 - D1)"=10, "Remote Source 0"=11, "Remote Source 1"=12, "Software Emulated"=15] ("Feedback Device")
            n288 = call <vilib>:"CTRE_Phoenix_MotorControl_ConfigSelectedFeedbackSensor_Enhanced.vi"("Feedback Device"=w492, "PhoenixMotorControlDevRef"=w493) -> ("PhoenixMotorControlDevRef"=w491:T12)  [unwired: 8 in, 1 out]
            n289 = call <vilib>:"CTRE_Phoenix_MotorControl_ConfigClosedLoopConstants.vi"("PhoenixMotorControlDevRef"=w491, "slotIdx"=0, "P"="P", "I"="I", "D"="D", "F"="kF", "I Zone"="I Zone") -> ("PhoenixMotorControlDevRef"=w483:T12)  [unwired: 7 in, 1 out]
            n290 = call-poly <vilib>:"CTRE_Phoenix_MotorController_Get_Enhanced.vi"("PhoenixMotorControlDevRef"=w483) -> ("Percent Output"=w477:dbl)  [unwired: 10 in, 4 out]
            "Voltage" <- w477
            n291 = call <vilib>:"CTRE_Phoenix_MotorControl_Set.vi"("Output"="FWSetpoint", "Control Mode"=w484, "PhoenixMotorControlDevRef"=w483) -> ()  [unwired: 7 in, 2 out]
            n292 = call-poly <vilib>:"CTRE_Phoenix_MotorController_Get_Enhanced.vi"("PhoenixMotorControlDevRef"=w483, "pidLoopIdx"=u32 0) -> ("Velocity (Raw Sensor Units per 100 ms)"=w480:i32)  [unwired: 10 in, 3 out]
            n293 = Bundle("FWSetpoint"="FWSetpoint", "Velocity (Raw Sensor Units per 100 ms)"=w480) -> (→"Velocity PIDF":T3)  [unwired: 1 in]
            n294 = Bundle("Percent Output"=w477) -> (→"Voltage Output":cluster{"Percent Output":dbl})  [unwired: 1 in]
          }
        }
        n295 = Wait (ms)(milliseconds to wait=u32 10) -> ()  [unwired: 1 out]
      }
    }
    frame Enabled {
    }
  }
  n296 = while {
    stop <- FALSE stop-if-true
    # "Distance by Limelight"
    n297 = global read "MotorsGlobal.vi" "LimelightY"() -> (w494:dbl)
    n298 = Add(x="Camera Angle", y=w494) -> (x+y=w496:dbl)
    n299 = expression code="(x/180.0)*pi" "degrees to radians"(w496) -> (w497:dbl)
    n300 = Subtract(x="Inner Goal Height", y="Camera Height") -> (x-y=w503:dbl)
    n301 = Tangent(1:w497) -> (0:w504:dbl)
    n302 = Divide(x=w503, y=w504) -> (x/y=→"Distancia do Goal":dbl)
    n303 = Wait (ms)(milliseconds to wait=u32 10) -> ()  [unwired: 1 out]
  }
